vi "AutoAlign_N664.vi"() -> ()   [LabVIEW 2014]
uses:
  Controls/StageStates.ctl
  Controls/GraphNotifier2D.ctl
panel:
  out "Current Step":i32
  in  "Done":bool
  in  "Repeat":bool
  in  "Start":bool
  out "Cursor Position":dbl=14.501547540983607
  in  "InitialStep":dbl=-0.5
  in  "StepSize":dbl=0.03
  in  "Number Of Steps":i32=35
  out "Intensity Graph":sgl[][](graph)=[[1575.0, 1530.0, 1467.0, 1650.0, 1682.0, 1613.0, 1536.0, 1626.0, 1940.0, 1831.0, 1587.0, 1388.0, 1511.0, 1435.0, 1379.0], [1709.0, 1679.0, 1771.0, 1769.0, 1775.0, 2008.0, 1804.0, 1975.0, 1770.0, 1847.0, 1595.0, 1554.0, 1478.0, 1427.0, 1513.0], [1648.0, 1736.0, 1646.0, 1749.0, 2076.0, 2140.0, 2064.0, 2285.0, 2553.0, 2003.0, 1778.0, 1592.0, 1374.0, 1409.0, 1484.0], [1691.0, 1662.0, 1787.0, 2129.0, 1967.0, 2135.0, 2802.0, 2654.0, 2620.0, 2152.0, 1653.0, 1625.0, 1294.0, 1626.0, 1484.0], [1791.0, 1866.0, 1955.0, 1940.0, 3130.0, 6076.0, 7812.0, 6999.0, 4445.0, 2270.0, 2108.0, 1656.0, 1663.0, 1432.0, 1434.0], [1685.0, 1692.0, 2032.0, 2360.0, 5595.0, 13786.0, 21952.0, 19970.0, 9456.0, 3969.0, 1980.0, 1953.0, 1670.0, 1777.0, 1482.0], [1690.0, 1883.0, 2231.0, 2992.0, 7277.0, 21162.0, 37225.0, 33877.0, 17031.0, 5558.0, 2486.0, 1757.0, 1705.0, 1721.0, 1629.0], [1950.0, 2070.0, 2444.0, 3114.0, 7300.0, 21633.0, 35295.0, 34230.0, 18542.0, 5857.0, 2447.0, 2046.0, 1718.0, 1496.0, 1497.0], [1738.0, 1911.0, 2271.0, 3013.0, 4517.0, 11402.0, 20736.0, 20231.0, 11390.0, 4490.0, 2670.0, 2143.0, 1981.0, 1468.0, 1542.0], [1875.0, 1741.0, 2051.0, 2522.0, 2677.0, 4632.0, 7218.0, 8580.0, 5418.0, 3381.0, 2550.0, 2068.0, 1621.0, 1690.0, 1591.0], [1727.0, 1602.0, 1790.0, 2337.0, 2453.0, 2325.0, 3198.0, 3570.0, 2998.0, 2777.0, 2034.0, 1844.0, 1659.0, 1637.0, 1530.0], [1562.0, 1616.0, 1920.0, 2051.0, 2025.0, 2333.0, 2346.0, 2577.0, 2301.0, 1999.0, 1878.0, 1700.0, 1628.0, 1624.0, 1486.0], [1599.0, 1666.0, 1677.0, 1735.0, 1646.0, 1710.0, 1950.0, 2008.0, 1755.0, 1922.0, 1644.0, 1723.0, 1616.0, 1341.0, 1659.0], [1496.0, 1555.0, 1749.0, 1781.0, 1666.0, 1880.0, 1703.0, 1865.0, 1750.0, 1712.0, 1685.0, 1646.0, 1592.0, 1380.0, 1439.0], [1706.0, 1543.0, 1659.0, 1490.0, 1552.0, 1610.0, 1653.0, 1799.0, 1670.0, 1665.0, 1578.0, 1393.0, 1625.0, 1681.0, 1501.0]]
  in  "Quit":bool
  out "Sample":cluster{"X":dbl, "Y":dbl}[](graph)
  in  "Accumulations":i32=10
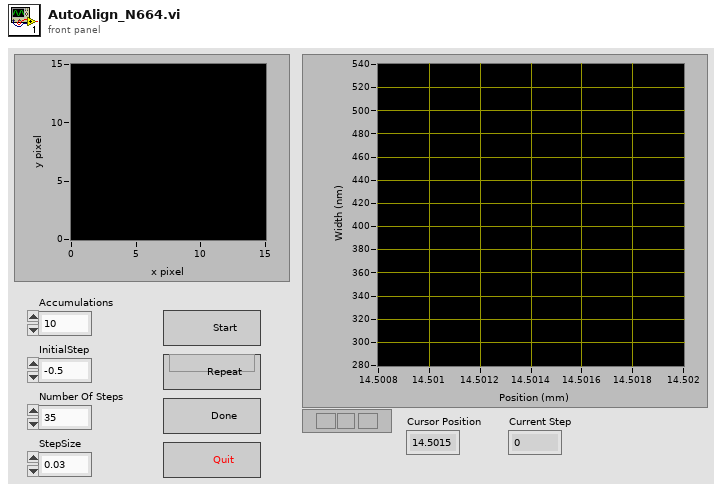
[diagram p1: front panel]
types:
  T1 = typedef "GraphNotifier2D.ctl" = cluster{"Xpos":i32, "Ypos":i32, "subarray":sgl[][], "Intensity":sgl}
  T2 = typedef "LabVIEW Interface for Arduino.lvlib/Arduino Resource.ctl" = cluster{"VISA resource":refnum<visa-resource-name>, "Board Type":T3, "Connection Type":enum8{"USB / Serial"}, "Bytes Per Packet (15)":u8}
  T3 = typedef "LabVIEW Interface for Arduino.lvlib/Board Type.ctl" = enum16{"Uno", "Dimuelanove w/Atmega 328", "Mega 2560"}
  T4 = typedef "StageStates.ctl" = enum16{"POSITION", "MVR", "MOVE", "HALT", "ONTARGET", "ERROR", "EXIT", "HOME", "ZEROPOS", "NANOPOS", "QUIT", "ANALOG"}
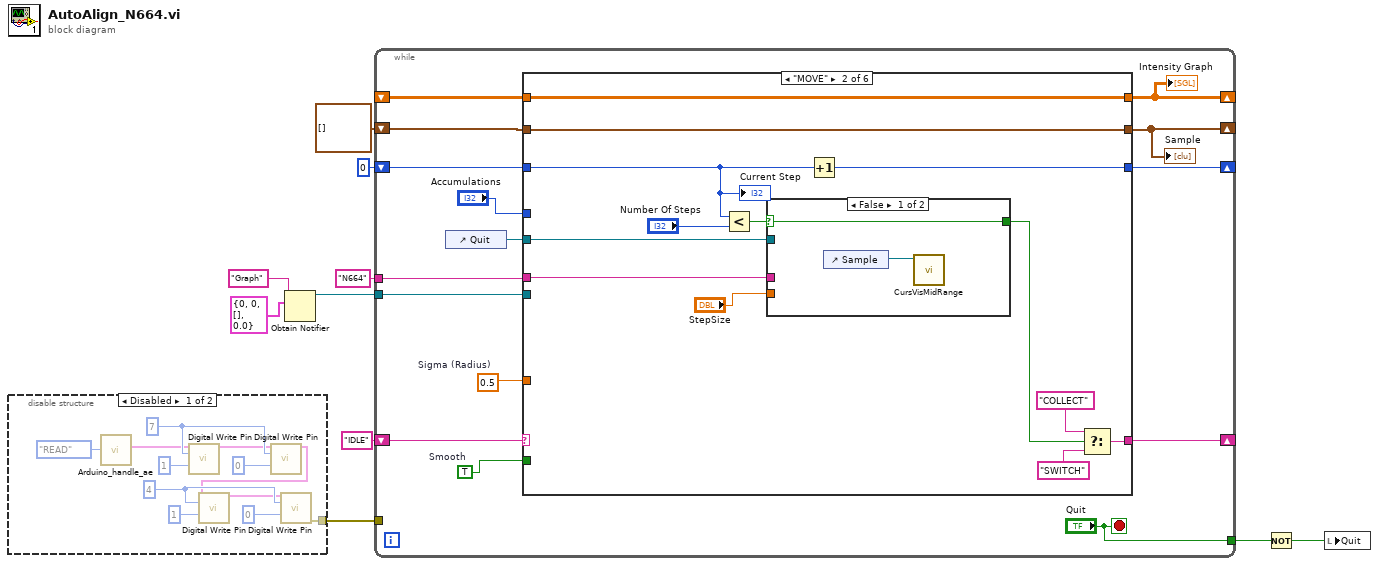
[diagram p0: block diagram]
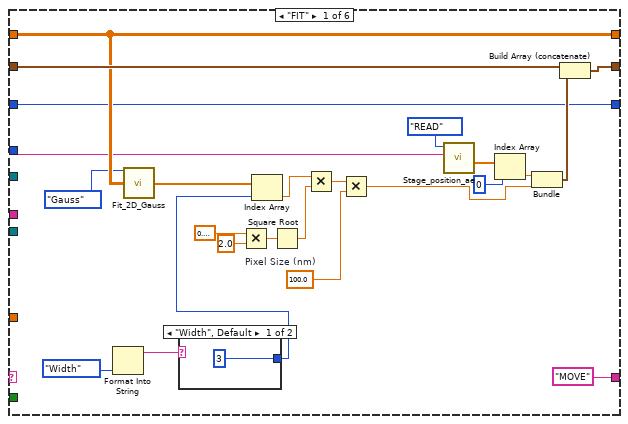
[diagram p3: hidden frame]
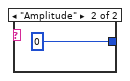
[diagram p4: hidden frame]
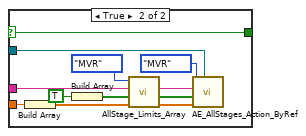
[diagram p5: hidden frame]
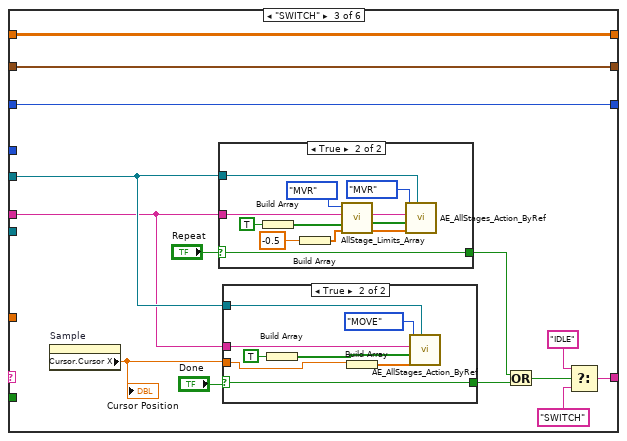
[diagram p6: hidden frame]
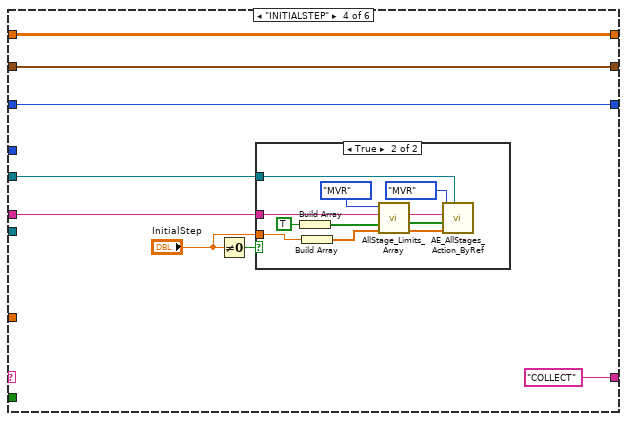
[diagram p9: hidden frame]
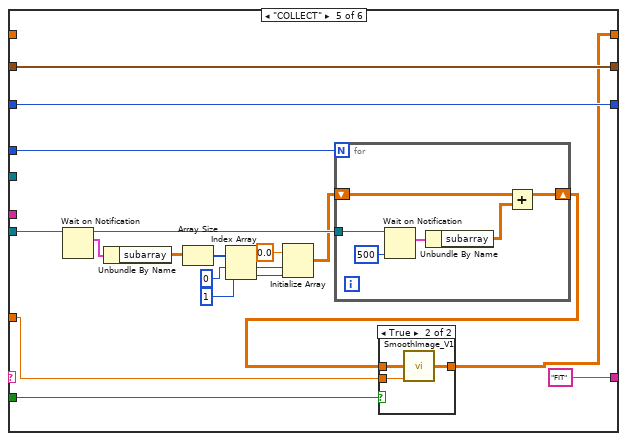
[diagram p11: hidden frame]
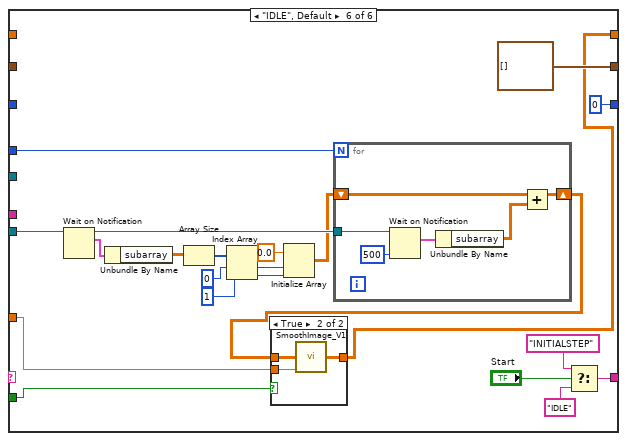
[diagram p13: hidden frame]
diagram:
  n1 = disable-structure shown="Disabled" {
    disable-tunnel: [w11 _] -> w6
    frame Disabled {
      w22 = u8 4 ("Digital I/O Pin (0)")
      w17 = u8 7 ("Digital I/O Pin (0)")
      n2 = call "Arduino_handle_ae.vi"("Enum"=enum16{"WRITE", "READ"}."READ") -> ("Arduino Resource Out"=w16:T2)  [unwired: 10 in]
      n3 = call <vilib>:"Digital Write Pin.vi"("Arduino Resource"=w16, "Digital I/O Pin (0)"=w17, "Value (0)"=u8 1) -> ("Arduino Resource"=w12:T2)  [unwired: 11 in, 1 out]
      n4 = call <vilib>:"Digital Write Pin.vi"("Arduino Resource"=w12, "Digital I/O Pin (0)"=w17, "Value (0)"=u8 0) -> ("Arduino Resource"=w21:T2)  [unwired: 11 in, 1 out]
      n5 = call <vilib>:"Digital Write Pin.vi"("Arduino Resource"=w21, "Digital I/O Pin (0)"=w22, "Value (0)"=u8 1) -> ("Arduino Resource"=w20:T2)  [unwired: 11 in, 1 out]
      n6 = call <vilib>:"Digital Write Pin.vi"("Arduino Resource"=w20, "Digital I/O Pin (0)"=w22, "Value (0)"=u8 0) -> ("error out"=w11:errorcluster)  [unwired: 11 in, 1 out]
    }
    frame Enabled {
    }
  }
  n7 = Obtain Notifier(name (unnamed)="Graph", notification data type=T1 {"Xpos"=0, "Ypos"=0, "subarray"=[], "Intensity"=0.0}) -> (notifier out=w3:refnum<notifier>)  [unwired: 2 in, 2 out]
  n8 = while {
    shift-right: [w35] -> _
    shift-left: _ -> [w37]
    shift-right: [w36] -> _
    shift-left: cluster{"x":dbl, "y":dbl}[] [] ("XY chart data") -> [w26]
    shift-right: [w34] -> _
    shift-left: "IDLE" -> [w30]
    shift-right: [w32] -> _
    shift-left: 0 ("NumberOfSteps 2") -> [w33]
    tunnel: w3 -> [w29]
    tunnel: "N664" ("StageID") -> [w27]
    tunnel: w6 -> [_]
    tunnel: ["Quit"] -> w2
    stop <- "Quit" stop-if-true
    w24 = 0.5  # Sigma (Radius)
    w23 = TRUE  # Smooth
    n9 = control-ref of="Quit"() -> (w31:refnum<vi>)
    n10 = case shown="\"MOVE\"" w30 {
      tunnel: [w57 w76 w102 w134 w148 w175] -> w35
      tunnel: w37 -> [w57 w76 w102 w134 _ _]
      tunnel: w26 -> [w59 w67 w103 w129 w164 _]
      tunnel: [w58 w67 w103 w129 w164 cluster{"x":dbl, "y":dbl}[] [] ("XY chart data")] -> w36
      tunnel: w27 -> [w54 w66 w99 w130 _ _]
      tunnel: ["MOVE" w73 w96 "COLLECT" "FIT" w195] -> w34
      tunnel: w33 -> [w55 w71 w104 w133 w163 _]
      tunnel: [w55 w72 w104 w133 w163 0 ("NumberOfSteps 2")] -> w32
      tunnel: w31 -> [_ w69 w101 w132 _ _]
      tunnel: w29 -> [_ _ _ _ w152 w188]
      tunnel: "Accumulations" -> [_ _ _ _ w161 w192]
      tunnel: w24 -> [_ _ _ _ w147 w177]
      tunnel: w23 -> [_ _ _ _ w146 w178]
      frame "FIT" {
        w47 = 100.0  # Pixel Size (nm)
        n11 = Format Into String(enum16{"Amplitude", "Width"}."Width" ("Fit parameter")) -> (resulting string=w40:string)  [unwired: 3 in, 1 out]
        n12 = call "Fit_2D_Gauss.vi"("Enum"=enum16{"Gauss", "Lorentz"}."Gauss", "Image IN"=w57) -> ("Fit Parameters"=w61:dbl[])  [unwired: 12 in, 1 out]
        n13 = case shown="\"Width\", Default" w40 {
          tunnel: [3 ("index") 0 ("index")] -> w39
          frame "Width", Default {
          }
          frame "Amplitude" {
          }
        }
        n14 = Multiply(x=0.6931471805599453, y=2.0) -> (x*y=w50:dbl)
        n15 = Index Array(array=w61, index=w39) -> (element=w48:dbl)
        n16 = Square Root(x=w50) -> (sqrt(x)=w53:dbl)
        n17 = Multiply(x=w48, y=w53) -> (x*y=w49:dbl)
        n18 = Multiply(x=w49, y=w47) -> (x*y=w42:dbl)
        n19 = call "Stage_position_ae.vi"("StageID"=w54, "Enum"=enum16{"WRITE", "READ"}."READ") -> ("Position Out"=w45:dbl[])  [unwired: 8 in, 1 out]
        n20 = Index Array(array=w45, index=0) -> (element=w43:dbl)
        n21 = Bundle("Numeric"=w43, w42) -> (w60:cluster{"Numeric":dbl, dbl})  [unwired: 1 in]
        n22 = Build Array (concatenate)(w59, w60) -> (w58:cluster{"Numeric":dbl, "y":dbl}[])
      }
      frame "MOVE" {
        n23 = Less?(x=w71, y="Number Of Steps") -> (x < y?=w64:bool)
        n24 = case shown="False" w64 {
          selector: w64 -> [w78 w87]
          tunnel: w66 -> [_ w82]
          tunnel: w69 -> [_ w88]
          tunnel: [w78 w87] -> w70
          tunnel: "StepSize" -> [_ w80]
          frame False {
            n25 = control-ref of="Sample"() -> (w77:refnum<vi>)
            n26 = call "CursVisMidRange.vi"("XYGraph in"=w77) -> ()  [unwired: 11 in]
          }
          frame True {
            n27 = Build Array(w80) -> (w79:dbl[])
            n28 = Build Array(TRUE) -> (w83:bool[])
            n29 = call "AllStage_Limits_Array.vi"("Step(um)/Position(units)"=w79, "Axis"=w83, "Stage ID"=w82, "MOVE/MVR"=enum16{"MOVE", "MVR"}."MVR") -> ("Positions"=w84:dbl[], "Boolean Array"=w85:bool[], "Stage ID"=w86:string)  [unwired: 5 in]
            n30 = call "AE_AllStages_Action_ByRef.vi"("Abort"=w88, "Positions"=w84, "Axis"=w85, "Stage ID"=w86, "Action"=StageStates."MVR") -> ()  [unwired: 3 in, 4 out]
          }
        }
        n31 = Increment(x=w71) -> (x+1=w72:i32)
        n32 = Select(t="COLLECT", s=w70, f="SWITCH") -> (s? t:f=w73:string)
        "Current Step" <- w71
      }
      frame "SWITCH" {
        n33 = property on="Sample" class="XYGraph (strict)"() -> ("Cursor.Cursor X"=w100:dbl)  [unwired: 2 in, 2 out]
        "Cursor Position" <- w100
        n34 = case shown="True" "Repeat" {
          selector: "Repeat" -> [w114 w117]
          tunnel: w99 -> [_ w118]
          tunnel: w101 -> [_ w124]
          tunnel: [w114 w117] -> w92
          frame False {
          }
          frame True {
            n35 = Build Array(TRUE) -> (w123:bool[])
            n36 = Build Array(-0.5 ("Step(um)/Position(units)")) -> (w115:dbl[])
            n37 = call "AllStage_Limits_Array.vi"("Step(um)/Position(units)"=w115, "Axis"=w123, "Stage ID"=w118, "MOVE/MVR"=enum16{"MOVE", "MVR"}."MVR") -> ("Positions"=w120:dbl[], "Boolean Array"=w121:bool[], "Stage ID"=w122:string)  [unwired: 5 in]
            n38 = call "AE_AllStages_Action_ByRef.vi"("Abort"=w124, "Positions"=w120, "Axis"=w121, "Stage ID"=w122, "Action"=StageStates."MVR") -> ()  [unwired: 3 in, 4 out]
          }
        }
        n39 = case shown="True" "Done" {
          selector: "Done" -> [w105 w110]
          tunnel: w99 -> [_ w109]
          tunnel: w101 -> [_ w111]
          tunnel: w100 -> [_ w107]
          tunnel: [w105 w110] -> w91
          frame False {
          }
          frame True {
            n40 = Build Array(TRUE) -> (w108:bool[])
            n41 = Build Array(w107) -> (w106:dbl[])
            n42 = call "AE_AllStages_Action_ByRef.vi"("Abort"=w111, "Positions"=w106, "Axis"=w108, "Stage ID"=w109, "Action"=StageStates."MOVE") -> ()  [unwired: 3 in, 4 out]
          }
        }
        n43 = Or(x=w92, y=w91) -> (x .or. y?=w95:bool)
        n44 = Select(t="IDLE", s=w95, f="SWITCH") -> (s? t:f=w96:string)
      }
      frame "INITIALSTEP" {
        n45 = Not Equal To 0?(x="InitialStep") -> (x != 0?=w128:bool)
        n46 = case shown="True" w128 {
          tunnel: w130 -> [_ w141]
          tunnel: w132 -> [_ w143]
          tunnel: "InitialStep" -> [_ w142]
          frame False {
          }
          frame True {
            n47 = Build Array(TRUE) -> (w139:bool[])
            n48 = Build Array(w142) -> (w135:dbl[])
            n49 = call "AllStage_Limits_Array.vi"("Step(um)/Position(units)"=w135, "Axis"=w139, "Stage ID"=w141, "MOVE/MVR"=enum16{"MOVE", "MVR"}."MVR") -> ("Positions"=w136:dbl[], "Boolean Array"=w137:bool[], "Stage ID"=w138:string)  [unwired: 5 in]
            n50 = call "AE_AllStages_Action_ByRef.vi"("Abort"=w143, "Positions"=w136, "Axis"=w137, "Stage ID"=w138, "Action"=StageStates."MVR") -> ()  [unwired: 3 in, 4 out]
          }
        }
      }
      frame "COLLECT" {
        n51 = Wait on Notification(notifier=w152) -> (notifier out=w151:refnum<notifier>, notification=w160:T1)  [unwired: 3 in, 2 out]
        n52 = Unbundle By Name(w160) -> ("subarray"=w159:sgl[][])
        n53 = Array Size(array=w159) -> (size(s)=w158:i32[])
        n54 = Index Array(array=w158, index #1=0 ("index"), index #2=1 ("index")) -> (element #1=w155:i32, element #2=w154:i32)
        n55 = Initialize Array(sgl 0.0 ("element"), w155, w154) -> (w150:sgl[][])
        n56 = for {
          N: w161 -> [_]
          shift-right: [w174] -> w149
          shift-left: w150 -> [w173]
          tunnel: w151 -> [w171]
          n57 = Wait on Notification(notifier=w171, timeout in ms (-1)=500) -> (notification=w170:T1)  [unwired: 2 in, 3 out]
          n58 = Unbundle By Name(w170) -> ("subarray"=w169:sgl[][])
          n59 = Add(x=w173, y=w169) -> (x+y=w174:sgl[][])
        }
        n60 = case shown="True" w146 {
          tunnel: w149 -> [w165 w168]
          tunnel: [w165 w167] -> w148
          tunnel: w147 -> [_ w166]
          frame False {
          }
          frame True {
            n61 = call "SmoothImage_V1.vi"("Image IN"=w168, "Sigma (Radius)"=w166) -> ("Smoothed Image"=w167:sgl[][])  [unwired: 13 in]
          }
        }
      }
      frame "IDLE", Default {
        n62 = Wait on Notification(notifier=w188) -> (notifier out=w187:refnum<notifier>, notification=w190:T1)  [unwired: 3 in, 2 out]
        n63 = Unbundle By Name(w190) -> ("subarray"=w189:sgl[][])
        n64 = Array Size(array=w189) -> (size(s)=w186:i32[])
        n65 = Index Array(array=w186, index #1=0 ("index"), index #2=1 ("index")) -> (element #1=w183:i32, element #2=w182:i32)
        n66 = Initialize Array(sgl 0.0 ("element"), w183, w182) -> (w180:sgl[][])
        n67 = for {
          N: w192 -> [_]
          shift-right: [w206] -> w176
          shift-left: w180 -> [w205]
          tunnel: w187 -> [w203]
          n68 = Wait on Notification(notifier=w203, timeout in ms (-1)=500) -> (notification=w202:T1)  [unwired: 2 in, 3 out]
          n69 = Unbundle By Name(w202) -> ("subarray"=w201:sgl[][])
          n70 = Add(x=w205, y=w201) -> (x+y=w206:sgl[][])
        }
        n71 = case shown="True" w178 {
          tunnel: w176 -> [w197 w200]
          tunnel: [w197 w199] -> w175
          tunnel: w177 -> [_ w198]
          frame False {
          }
          frame True {
            n72 = call "SmoothImage_V1.vi"("Image IN"=w200, "Sigma (Radius)"=w198) -> ("Smoothed Image"=w199:sgl[][])  [unwired: 13 in]
          }
        }
        n73 = Select(t="INITIALSTEP", s="Start", f="IDLE") -> (s? t:f=w195:string)
      }
    }
    "Sample" <- w36
    "Intensity Graph" <- w35
  }
  n74 = Not(x=w2) -> (.not. x?=w1:bool)
  n75 = local write "Quit"(w1) -> ()
